vi "Cleanup Instrument Engine.vi"(8 "error in (no error)":errorcluster, 11 "State Variables":T1) -> ()   [LabVIEW 2019, in "Instrument Addon Engine.lvlib"]
uses:
  Instrument Addon Engine.lvlib
  Types/Engine State Variables.ctl
  <vilib>/NI/NIVS Inline Async API/_VS Inline Async API/Process/Process.lvclass
  <vilib>/NI/NIVS Addon Network Comm/Engine/VeriStand Comm.lvclass
  <vilib>/NI/NIVS Inline Async API/_Data Access Engine/Data Access Engine/Types/Write.DVR.ctl
  <vilib>/NI/NIVS Inline Async API/_Data Access Engine/Access Type Classes/Write/Write.lvclass
  <vilib>/NI/NIVS Inline Async API/_Data Access Engine/Data Access Engine/Types/Read.DVR.ctl
  <vilib>/NI/NIVS Inline Async API/_Data Access Engine/Access Type Classes/Read/Read.lvclass
  <vilib>/NI/NIVS Inline Async API/_Data Access Engine/Data Access Engine/Types/ReadWrite.DVR.ctl
  <vilib>/NI/NIVS Inline Async API/_Data Access Engine/Access Type Classes/ReadWrite/ReadWrite.lvclass
  <vilib>/NI VeriStand/Custom Device Tools/Custom Device Utility Library/Custom Device Utility Library.lvlib
  <vilib>/NI/NIVS Inline Async API/_Data Access Engine/Data Access Engine/Data Access Engine.lvclass
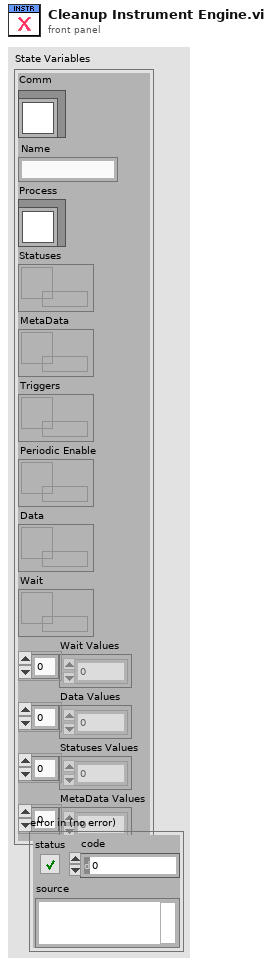
[diagram p1: front panel]
types:
  T1 = typedef "Instrument Addon Engine.lvlib/Engine State Variables.ctl" = cluster{"Comm":refnum<class "VeriStand Comm.lvclass">, "Name":string, "Process":refnum<class "Process.lvclass">, "Statuses":T2, "MetaData":T3, "Triggers":T4, "Periodic Enable":T3, "Data":T2, "Wait":T3, "Wait Values":dbl[], "Data Values":dbl[], "Statuses Values":dbl[], "MetaData Values":dbl[]}
  T2 = typedef "Data Access Engine.lvlib/Data Access Engine.lvclass/Write.DVR.ctl" = refnum<data-value>
  T3 = typedef "Data Access Engine.lvlib/Data Access Engine.lvclass/Read.DVR.ctl" = refnum<data-value>
  T4 = typedef "Data Access Engine.lvlib/Data Access Engine.lvclass/ReadWrite.DVR.ctl" = refnum<data-value>
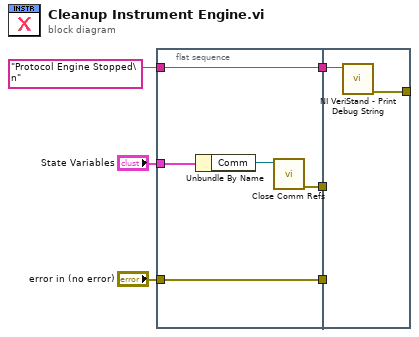
[diagram p0: block diagram]
diagram:
  n1 = flat-sequence {
    tunnel: "error in (no error)" -> [w8]
    tunnel: "Protocol Engine Stopped\n" ("Debug String") -> [w10]
    tunnel: "State Variables" -> [w11]
    tunnel: [w10] -> w6
    tunnel: [w9] -> w5
    tunnel: [w8] -> w1
    tunnel: w6 -> [w12]
    tunnel: w5 -> [_]
    tunnel: w1 -> [_]
    tunnel: [w13] -> _
    frame #0 {
      n2 = Unbundle By Name(w11) -> ("Comm"=w7:refnum<class "VeriStand Comm.lvclass">)
      n3 = call <vilib>:"Close Comm Refs.vi"("Comm.lvclass"=w7) -> ("error out"=w9:errorcluster)  [unwired: 10 in]
    }
    frame #1 {
      n4 = call <vilib>:"NI VeriStand - Print Debug String.vi"("Message"=w12) -> ("error out"=w13:errorcluster)  [unwired: 10 in]
    }
  }
